vi "Load Steps.vi"(6 "Constants":refnum<class "Sequence Constants.lvclass">, 8 "error in":refnum<class "MultiErrors.lvclass">, 10 "Config Element":refnum<class "Config Element.lvclass">) -> (0 "error out":refnum<class "MultiErrors.lvclass">, 2 "Steps":T1[](array[typedef]))   [LabVIEW 2020, in "VolatusSeqConfig.lvlib" / "Sequence Config.lvclass"]
uses:
  Sequence Config.lvclass
  lv-cdm/CDM-Config/Config Element/Config Element.lvclass
  Step.ctl
  Command Config/Command Config.lvclass
  VolatusErrorUtilities/MultiErrors/MultiErrors.lvclass
  VolatusErrorUtilities/MultiErrors/MultiErrors.lvclass/MultiErrors.ctl
  Sequence Config.lvclass/Sequence Config.ctl
  VolatusSeqConfig.lvlib
  Sequence Constants/Sequence Constants.lvclass
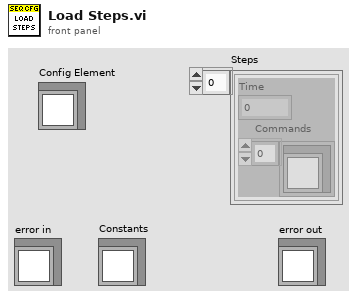
[diagram p1: front panel]
types:
  T1 = typedef "VolatusSeqConfig.lvlib/Step.ctl" = cluster{"Time":dbl, "Commands":refnum<class "Command Config.lvclass">[]}
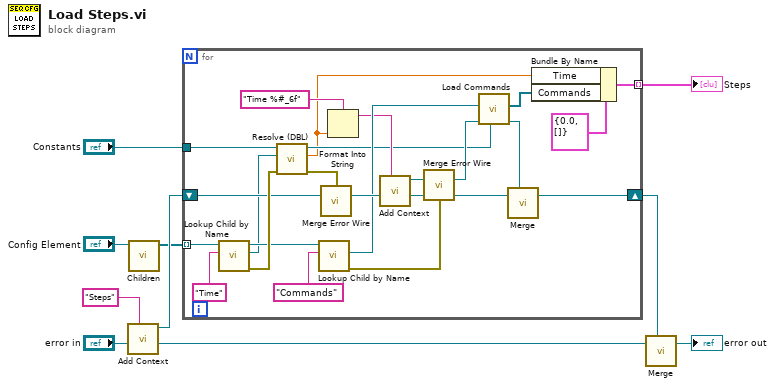
[diagram p0: block diagram]
diagram:
  n1 = call "Add Context.vi"("Context"="Steps", "MultiErrors in"="error in") -> ("Original Context"=w4:refnum<class "MultiErrors.lvclass">, "Added Context"=w10:refnum<class "MultiErrors.lvclass">)  [unwired: 8 in]
  n2 = call "Children.vi"("Config Element in"="Config Element") -> ("Elements"=w8:refnum<class "Config Element.lvclass">[])  [unwired: 9 in, 1 out]
  n3 = for {
    tunnel: w8 -> [w30] mode=indexing
    tunnel: [w27] -> w7 mode=indexing
    shift-right: [w20] -> w3
    shift-left: w10 -> [w31]
    tunnel: "Constants" -> [w15]
    n4 = call "Lookup Child by Name.vi"("Name"="Time", "Config Element in"=w30) -> ("error out"=w34:errorcluster, "Child"=w12:refnum<class "Config Element.lvclass">, "Config Element out"=w26:refnum<class "Config Element.lvclass">)  [unwired: 6 in, 1 out]
    n5 = call "Resolve (DBL).vi"("error in (no error)"=w34, "Element"=w12, "Sequence Constants in"=w15) -> ("error out"=w13:errorcluster, "DBL Value"=w11:dbl, "Sequence Constants out"=w14:refnum<class "Sequence Constants.lvclass">)  [unwired: 6 in]
    n6 = call "Lookup Child by Name.vi"("Name"="Commands", "Config Element in"=w26) -> ("error out"=w32:errorcluster, "Child"=w24:refnum<class "Config Element.lvclass">)  [unwired: 6 in, 2 out]
    n7 = call "Merge Error Wire.vi"("error in (no error)"=w13, "MultiErrors in"=w31) -> ("MultiErrors out"=w33:refnum<class "MultiErrors.lvclass">)  [unwired: 13 in]
    n8 = Format Into String(format string="Time %#_6f", w11) -> (resulting string=w19:string)  [unwired: 2 in, 1 out]
    n9 = call "Add Context.vi"("Context"=w19, "MultiErrors in"=w33) -> ("Original Context"=w22:refnum<class "MultiErrors.lvclass">, "Added Context"=w17:refnum<class "MultiErrors.lvclass">)  [unwired: 8 in]
    n10 = call "Merge Error Wire.vi"("error in (no error)"=w32, "MultiErrors in"=w17) -> ("MultiErrors out"=w16:refnum<class "MultiErrors.lvclass">)  [unwired: 13 in]
    n11 = call "Load Commands.vi"("Constants"=w14, "error in"=w16, "Config Element"=w24) -> ("error out"=w21:refnum<class "MultiErrors.lvclass">, "Commands"=w23:refnum<class "Command Config.lvclass">[])  [unwired: 7 in]
    n12 = call "Merge.vi"("First Error In"=w22, "Second Error In"=w21) -> ("MultiErrors out"=w20:refnum<class "MultiErrors.lvclass">)  [unwired: 5 in]
    n13 = Bundle By Name(cluster=T1 {"Time"=0.0, "Commands"=[]} ("Step"), "Time"=w11, "Commands"=w23) -> (w27:T1)
  }
  "Steps" <- w7
  n14 = call "Merge.vi"("First Error In"=w4, "Second Error In"=w3) -> ("MultiErrors out"=→"error out":refnum<class "MultiErrors.lvclass">)  [unwired: 5 in]
